vi "Excel Get Data Specified Field String.vi"(4 "error in (no error)":errorcluster, 5 "SheetName":string="Sheet1", 6 "path":path, 7 "Start and End":T1) -> (0 "error out":errorcluster, 2 "data":string[][](array[string]))   [LabVIEW 2014]
panel:
  out "array 2":dbl[][](array[numeric])
  in  "Excel._Worksheet 2":refnum<k7>
  in  "Array":string[][](array[string])
  in  "Excel._Worksheet":refnum<k7>
  in  "Excel._Application":refnum<k7>
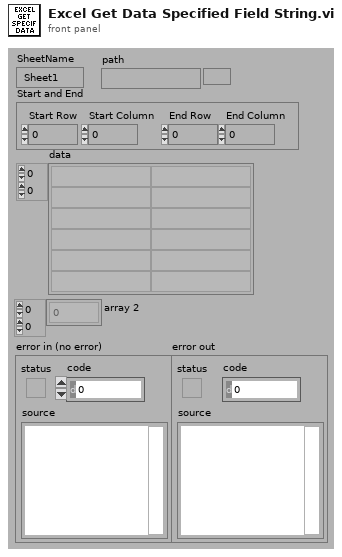
[diagram p1: front panel]
types:
  T1 = cluster{"Start Row":i32, "Start Column":i32, "End Row":i32, "End Column":i32}
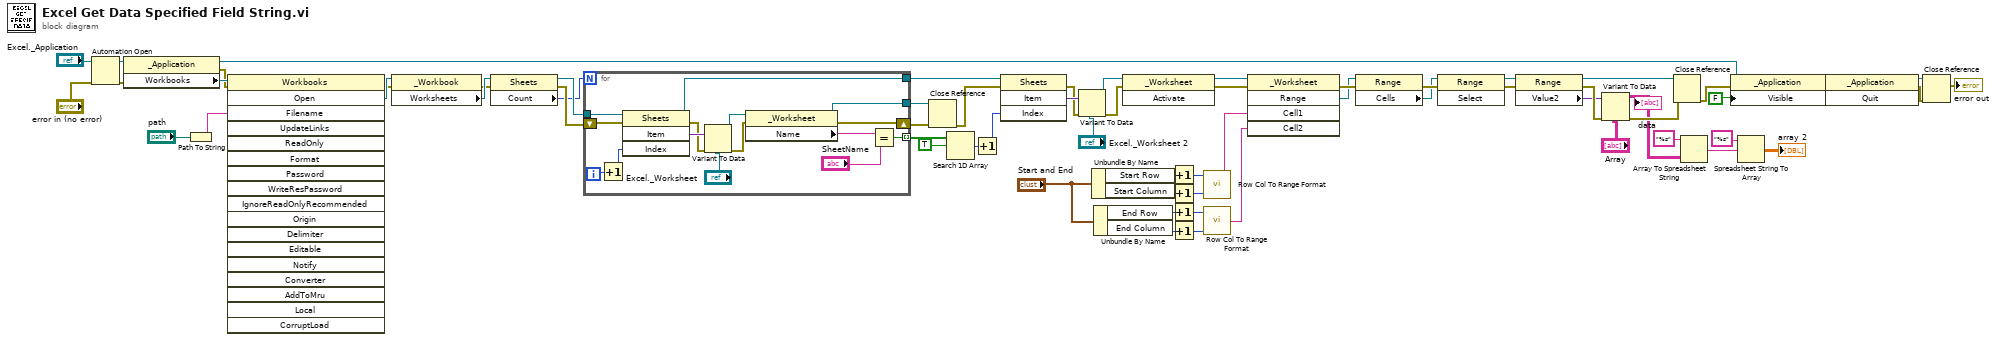
[diagram p0: block diagram]
diagram:
  n1 = Automation Open(error in (no error)="error in (no error)", Automation Refnum="Excel._Application") -> (Automation Refnum=w63:refnum<k7>, error out=w62:errorcluster)  [unwired: 2 in]
  n2 = property class="_Application"(reference=w63, error in=w62) -> (reference out=w53:refnum<k7>, error out=w56:errorcluster, "Workbooks"=w57:refnum<k7>)
  n3 = Path To String(path="path") -> (string=w3:string)
  n4 = invoke class="Workbooks" method="Open"(reference=w57, error in=w56, "Filename"=w3) -> (error out=w54:errorcluster, "Open"=w55:refnum<k7>)  [unwired: 15 in, 16 out]
  n5 = property class="_Workbook"(reference=w55, error in=w54) -> (error out=w41:errorcluster, "Worksheets"=w42:refnum<k7>)  [unwired: 1 out]
  n6 = property class="Sheets"(reference=w42, error in=w41) -> (reference out=w40:refnum<k7>, error out=w36:errorcluster, "Count"=w32:i32)
  n7 = for {
    N: w32 -> [_]
    tunnel: w40 -> [w80]
    shift-right: [w69] -> w31
    shift-left: w36 -> [w79]
    tunnel: [w70] -> w33 mode=indexing
    tunnel: [w68] -> w34
    tunnel: [w67] -> w29
    i -> [w77]
    n8 = Increment(x=w77) -> (x+1=w78:i32)
    n9 = invoke class="Sheets" method="Item"(reference=w80, error in=w79, "Index"=w78) -> (reference out=w68:refnum<k7>, error out=w74:errorcluster, "Item"=w76:variant)  [unwired: 1 in, 1 out]
    n10 = Variant To Data(error in=w74, type="Excel._Worksheet", Variant=w76) -> (data=w72:refnum<k7>, error out=w73:errorcluster)
    n11 = property class="_Worksheet"(reference=w72, error in=w73) -> (reference out=w67:refnum<k7>, error out=w69:errorcluster, "Name"=w71:string)
    n12 = Equal?(x=w71, y="SheetName") -> (x = y?=w70:bool)
  }
  n13 = Close Reference(reference=w29, error in (no error)=w31) -> (error out=w30:errorcluster)
  n14 = Search 1D Array(1D array=w33, element=TRUE) -> (index of element=w38:i32)  [unwired: 1 in]
  n15 = Increment(x=w38) -> (x+1=w37:i32)
  n16 = invoke class="Sheets" method="Item"(reference=w34, error in=w30, "Index"=w37) -> (error out=w60:errorcluster, "Item"=w61:variant)  [unwired: 1 in, 2 out]
  n17 = Variant To Data(error in=w60, type="Excel._Worksheet 2", Variant=w61) -> (data=w28:refnum<k7>, error out=w59:errorcluster)
  n18 = Unbundle By Name("Start and End") -> ("Start Row"=w14:i32, "Start Column"=w13:i32)
  n19 = Unbundle By Name("Start and End") -> ("End Row"=w12:i32, "End Column"=w11:i32)
  n20 = invoke class="_Worksheet" method="Activate"(reference=w28, error in=w59) -> (reference out=w19:refnum<k7>, error out=w18:errorcluster)  [unwired: 1 in, 1 out]
  n21 = Increment(x=w14) -> (x+1=w16:i32)
  n22 = Increment(x=w13) -> (x+1=w17:i32)
  n23 = Increment(x=w12) -> (x+1=w10:i32)
  n24 = Increment(x=w11) -> (x+1=w9:i32)
  n25 = call "Row Col To Range Format.vi"("Column"=w17, "Row"=w16) -> ("Output String"=w8:string)
  n26 = call "Row Col To Range Format.vi"("Column"=w9, "Row"=w10) -> ("Output String"=w7:string)
  n27 = invoke class="_Worksheet" method="Range"(reference=w19, error in=w18, "Cell1"=w8, "Cell2"=w7) -> (error out=w6:errorcluster, "Range"=w5:refnum<k7>)  [unwired: 1 in, 3 out]
  n28 = property class="Range"(reference=w5, error in=w6) -> (error out=w50:errorcluster, "Cells"=w27:refnum<k7>)  [unwired: 1 out]
  n29 = invoke class="Range" method="Select"(reference=w27, error in=w50) -> (reference out=w49:refnum<k7>, error out=w48:errorcluster)  [unwired: 1 in, 1 out]
  n30 = property class="Range"(reference=w49, error in=w48) -> (reference out=w46:refnum<k7>, error out=w47:errorcluster, "Value2"=w43:variant)
  n31 = Variant To Data(error in=w47, type="Array", Variant=w43) -> (data=w4:string[][], error out=w45:errorcluster)
  "data" <- w4
  n32 = Close Reference(reference=w46, error in (no error)=w45) -> (error out=w44:errorcluster)
  n33 = Array To Spreadsheet String(array=w4, 3:"%s" ("format string")) -> (spreadsheet string=w22:string)  [unwired: 1 in]
  n34 = property class="_Application"(reference=w53, error in=w44, "Visible"=FALSE) -> (reference out=w51:refnum<k7>, error out=w52:errorcluster)
  n35 = Spreadsheet String To Array(format string="%s", spreadsheet string=w22) -> (array=→"array 2":dbl[][])  [unwired: 2 in]
  n36 = invoke class="_Application" method="Quit"(reference=w51, error in=w52) -> (reference out=w26:refnum<k7>, error out=w25:errorcluster)  [unwired: 1 in, 1 out]
  n37 = Close Reference(reference=w26, error in (no error)=w25) -> (error out=→"error out":errorcluster)
